vi "Set Pin Infos.vi"(0 "Display State In":T3, 7 "Pin Info Array":T1, 9 "Container State":T4, 11 "error in (no error)":errorcluster) -> (4 "Display State Out":T3, 15 "error out":errorcluster)   [LabVIEW 2021, in "roboRIO 4 Bank.xctl"]
uses:
  <vilib>/myRIO/Common/Instrument Driver Framework/Utilities/xctls/roboRIO 4 Bank/roboRIO 4 Bank.xctl
  <vilib>/_xctls/Container State.ctl
  <vilib>/myRIO/Common/Instrument Driver Framework/Utilities/xctls/roboRIO 4 Bank/State.ctl
  <vilib>/myRIO/Common/Instrument Driver Framework/Utilities/xctls/utilities/typedefs/myRIOXC Pin Info Array.ctl
  <vilib>/myRIO/Common/Instrument Driver Framework/Utilities/xctls/utilities/typedefs/myRIOXC Pin Info.ctl
  <vilib>/myRIO/Common/Instrument Driver Framework/Utilities/xctls/utilities/vis/roboRIO Set Pin Info.vi
  <vilib>/_xctls/XControlSupport.lvlib
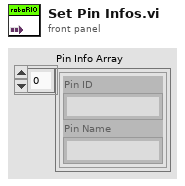
[diagram p1: front panel]
types:
  T1 = typedef "myRIOXC Pin Info Array.ctl" = T2[]
  T2 = typedef "myRIOXC Pin Info.ctl" = cluster{"Pin ID":string, "Pin Name":string}
  T3 = typedef "roboRIO 4 Bank.xctl/State.ctl" = cluster{"Pin Disabled?":enum8{"Enabled", "Disabled", "Disabled and Grayed Out"}[], "Pin Name":string[], "Pin ID":string[], "Connector Name":string, "Row Name 1":string, "Row Name 2":string}
  T4 = typedef "XControlSupport.lvlib/Container State.ctl" = cluster{"Indicator?":bool, "Run Mode?":bool, " Refnum":refnum<vi>}
  T5 = typedef "roboRIO Bank Display State.ctl" = cluster{"Pin Disabled?":enum8{"Enabled", "Disabled", "Disabled and Grayed Out"}[], "Pin Name":string[], "Pin ID":string[], "Connector Name":string, "Row Name 1":string, "Row Name 2":string}
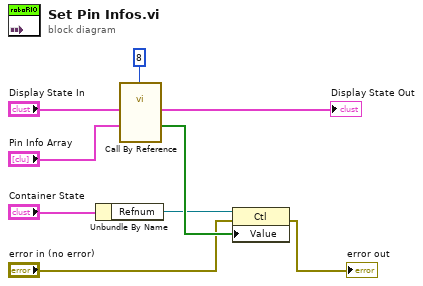
[diagram p0: block diagram]
diagram:
  n1 = Unbundle By Name("Container State") -> ("Refnum"=w5:refnum<vi>)
  n2 = call-by-ref "?"("Size"=8, "Pin Info Array"="Pin Info Array", "Display State In in"="Display State In") -> ("Data"=w6:bool[], "Display State In out"=→"Display State Out":T5)  [unwired: 9 in, 2 out]
  n3 = property class="Ctl"(reference=w5, error in="error in (no error)", "Value"=w6) -> (error out=→"error out":errorcluster)  [unwired: 1 out]
